vi "Delay with Stopwatch.vi"(4 "error in":errorcluster, 6 "window title":string="Waiting", 7 "delay":dbl[unit]=3.0 caption="Time Target (s)" format="%_3g") -> (0 "error out":errorcluster {"code" format="%.0x"})   [LabVIEW 2020]
panel:
  out "Stop 2":bool
  in  "stop":bool
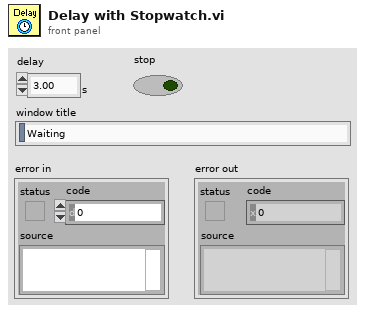
[diagram p1: front panel]
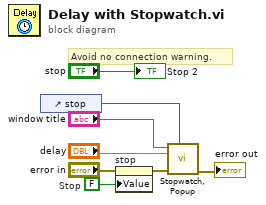
[diagram p0: block diagram]
diagram:
  w4 = FALSE  # Stop
  # "Avoid no connection warning."
  n1 = control-ref of="stop"() -> (w7:refnum<vi>)
  n2 = property on="stop" class="Bool (strict)"(error in="error in", "Value"=w4) -> (error out=w2:errorcluster)  [unwired: 1 in, 1 out]
  n3 = call "Stopwatch, Popup.vi"("Stop (Bool) Refnum"=w7, "error in (no error)"=w2, "Time Target"="delay", "Front Panel Window:Title"="window title") -> ("error out"=→"error out":errorcluster)  [unwired: 5 in, 2 out]
  "Stop 2" <- "stop"
